vi "Clear Scan Time Out_4.vi"(6 "Channel number":i32, 7 "ESP32 ref":refnum<visa-resource-name>="COM4", 8 "error in (no error)":errorcluster, 11 "VISA Refnum in":refnum<visa-resource-name>) -> (0 "error out":errorcluster, 1 "error?":bool, 2 "Time out count":i32, 3 "VISA Refnum out":refnum<visa-resource-name>, 5 "ESP32 ref out":refnum<visa-resource-name>)   [LabVIEW 2023]
uses:
  <vilib>/Utility/error.llb/DialogType.ctl
  <instrlib>/Agilent 3446X Series/Agilent 3446X Series.lvlib
panel:
  out "error out 3":errorcluster
  out "error out 2":errorcluster
  out "s? t:f 2":bool
  out "Measurements":dbl[](array[numeric])
  out "length":i32
  out "array":dbl[](array[numeric])
  out "return count":u32
  out "Channel number 2":i32
  out "size(s)":i32
  out "x >= y?":bool
  out "s? t:f":bool
  out "Numeric":i32
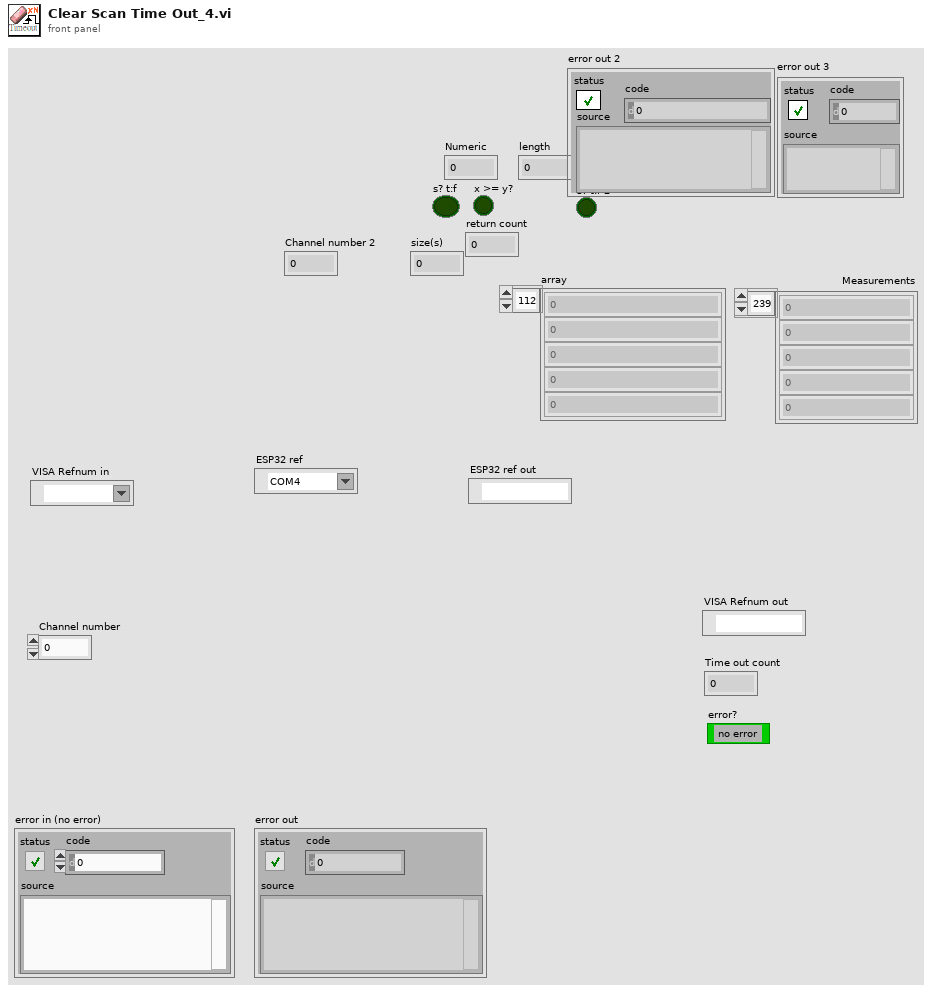
[diagram p1: front panel]
types:
  T1 = typedef "DialogType.ctl" = u16
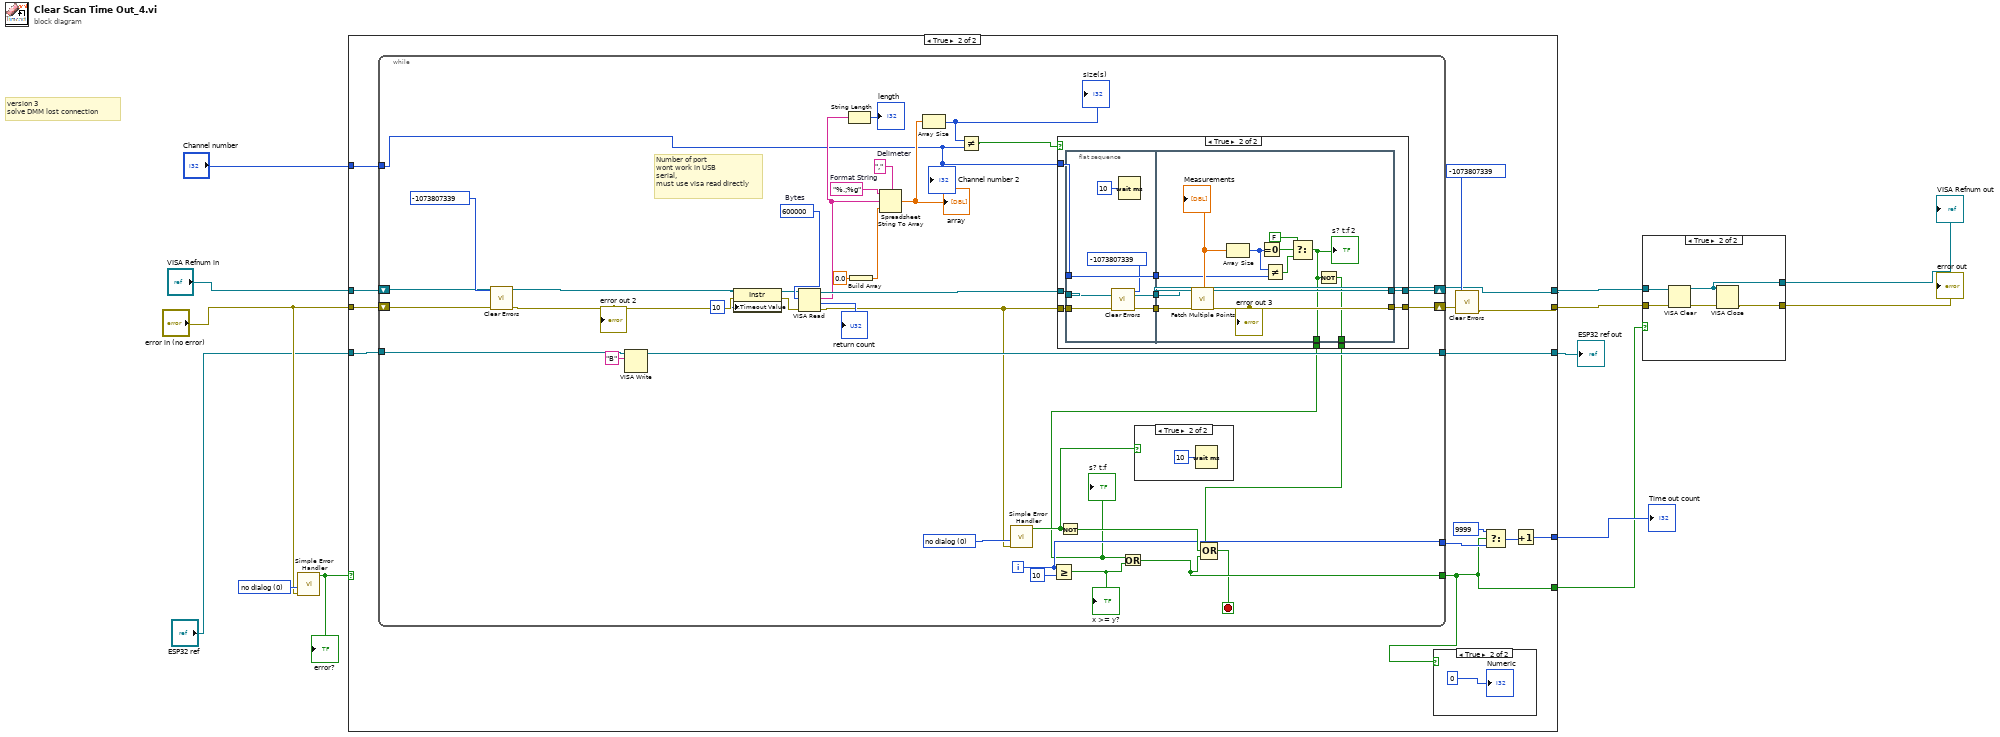
[diagram p0: block diagram]
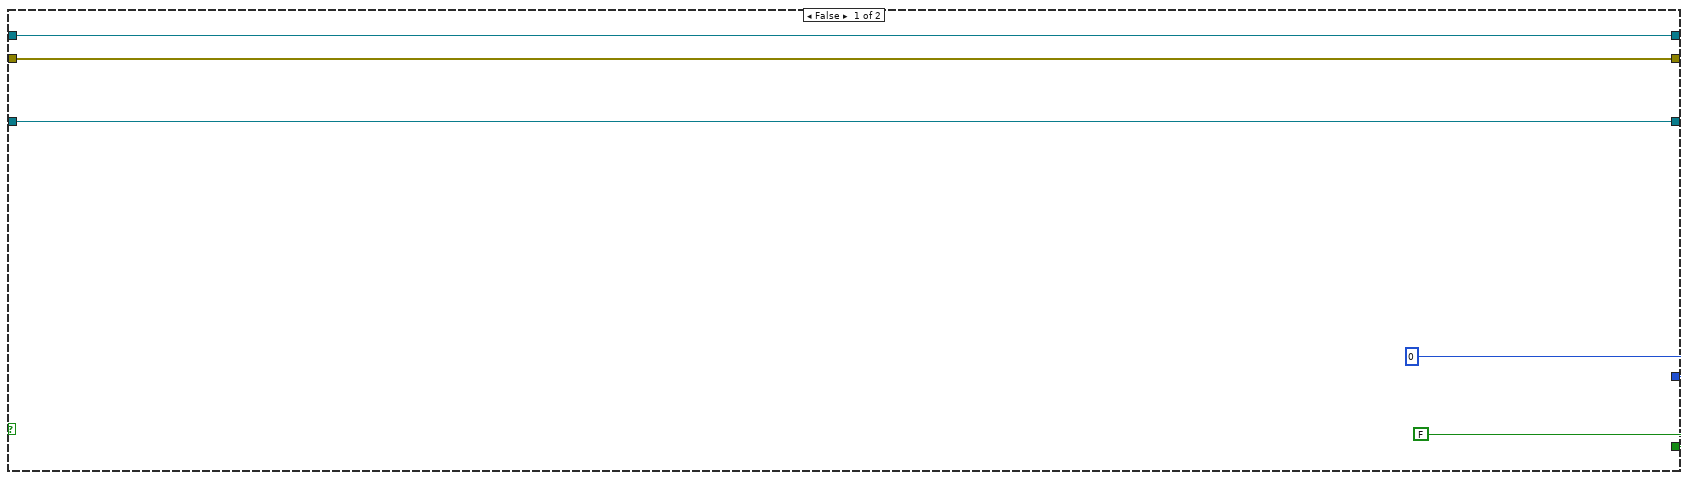
[diagram p3: hidden frame]
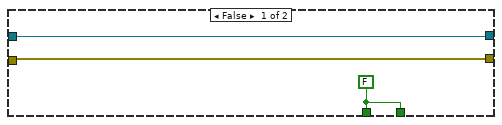
[diagram p5: hidden frame]
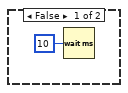
[diagram p6: hidden frame]
diagram:
  w12 = T1 0 items=["no dialog", "OK message", "continue or stop message", "OK message + warnings", "continue/stop + warnings"] ("type of dialog (OK msg:1)")
  # "version 3\nsolve DMM lost connection"
  n1 = call <vilib>:"Simple Error Handler.vi"("type of dialog (OK msg:1)"=w12, "error in (no error)"="error in (no error)") -> ("error?"=w10:bool)  [unwired: 3 in, 4 out]
  "error?" <- w10
  n2 = case shown="True" w10 {
    tunnel: [w18 w21] -> w4
    tunnel: "error in (no error)" -> [w17 w32]
    tunnel: "VISA Refnum in" -> [w18 w31]
    tunnel: [w17 w20] -> w3
    tunnel: [0 w30] -> w9
    tunnel: "ESP32 ref" -> [w16 w28]
    tunnel: [w16 w27] -> w7
    tunnel: "Channel number" -> [_ w26]
    tunnel: [FALSE w19] -> w5
    frame False {
    }
    frame True {
      n3 = while {
        shift-right: [w40] -> w25
        shift-left: w32 -> [w68]
        shift-right: [w41] -> w21
        shift-left: w31 -> [w53]
        tunnel: [w45] -> w22
        tunnel: [w49] -> w19
        tunnel: w28 -> [w52]
        tunnel: [w47] -> w27
        tunnel: w26 -> [w37]
        i -> [w45]
        stop <- w46 stop-if-true
        w60 = ","  # Delimeter
        w61 = "%.;%g"  # Format String
        w57 = u32 600000  # Bytes
        w66 = T1 0 items=["no dialog", "OK message", "continue or stop message", "OK message + warnings", "continue/stop + warnings"] ("type of dialog (OK msg:1)")
        # "Number of port\nwont work in USB \nserial,\nmust use visa read directly"
        n4 = call <vilib>:"Clear Errors.vi"("error in (no error)"=w68, "specific error code to clear (0: all)"=-1073807339 ("code out")) -> ("error out"=w67:errorcluster)  [unwired: 4 in, 1 out]
        "error out 2" <- w67
        n5 = VISA Write(VISA resource name=w52, write buffer="B") -> (VISA resource name out=w47:refnum<visa-resource-name>)  [unwired: 1 in, 2 out]
        n6 = property class="Instr"(reference=w53, error in=w67, "General Settings:Timeout Value"=u32 10) -> (reference out=w56:refnum<visa-resource-name>, error out=w55:errorcluster)
        n7 = VISA Read(VISA resource name=w56, byte count=w57, error in (no error)=w55) -> (VISA resource name out=w43:refnum<visa-resource-name>, read buffer=w39:string, return count=→"return count":u32, error out=w42:errorcluster)
        n8 = String Length(string=w39) -> (length=→"length":i32)
        n9 = Build Array(0.0) -> (w58:dbl[])
        n10 = Spreadsheet String To Array(delimiter (Tab)=w60, format string=w61, spreadsheet string=w39, array type (2D Dbl)=w58) -> (array=w51:dbl[])
        "array" <- w51
        n11 = Array Size(array=w51) -> (size(s)=w48:i32)
        "size(s)" <- w48
        n12 = Not Equal?(x=w48, y=w37) -> (x != y?=w34:bool)
        n13 = call <vilib>:"Simple Error Handler.vi"("type of dialog (OK msg:1)"=w66, "error in (no error)"=w42) -> ("error?"=w63:bool)  [unwired: 3 in, 4 out]
        n14 = Greater Or Equal?(x=w45, y=10) -> (x >= y?=w50:bool)
        "x >= y?" <- w50
        n15 = case shown="True" w34 {
          tunnel: w43 -> [w72 w79]
          tunnel: w42 -> [w71 w78]
          tunnel: [w72 w77] -> w41
          tunnel: [w71 w76] -> w40
          tunnel: w37 -> [_ w75]
          tunnel: [w70 w74] -> w36
          tunnel: [w70 w73] -> w35
          frame False {
            w70 = FALSE ("t")
          }
          frame True {
            n16 = flat-sequence {
              tunnel: w78 -> [w85]
              tunnel: w79 -> [w88]
              tunnel: [w88] -> w82
              tunnel: [w84] -> w81
              tunnel: w75 -> [w86]
              tunnel: [w86] -> w80
              tunnel: [w98] -> w77
              tunnel: [w97] -> w76
              tunnel: w82 -> [w100]
              tunnel: w81 -> [w99]
              tunnel: w80 -> [w91]
              tunnel: [w90] -> w74
              tunnel: [w89] -> w73
              frame #0 {
                n17 = call <vilib>:"Clear Errors.vi"("error in (no error)"=w85, "specific error code to clear (0: all)"=-1073807339) -> ("error out"=w84:errorcluster)  [unwired: 4 in, 1 out]
                n18 = Wait (ms)(milliseconds to wait=u32 10) -> ()  [unwired: 1 out]
              }
              frame #1 {
                n19 = call <instrlib>:"Fetch Multiple Points.vi"("error in (no error)"=w99, "VISA resource name"=w100) -> ("error out"=w97:errorcluster, "Measurements"=w92:dbl[], "VISA resource name out"=w98:refnum<visa-resource-name>)  [unwired: 7 in]
                "Measurements" <- w92
                "error out 3" <- w97
                n20 = Array Size(array=w92) -> (size(s)=w93:i32)
                n21 = Equal To 0?(x=w93) -> (x = 0?=w96:bool)
                n22 = Not Equal?(x=w93, y=w91) -> (x != y?=w95:bool)
                n23 = Select(t=FALSE, s=w96, f=w95) -> (s? t:f=w90:bool)
                "s? t:f 2" <- w90
                n24 = Not(x=w90) -> (.not. x?=w89:bool)
              }
            }
          }
        }
        "s? t:f" <- w36
        n25 = Not(x=w63) -> (.not. x?=w64:bool)
        n26 = Or(x=w36, y=w50) -> (x .or. y?=w49:bool)
        n27 = case shown="True" w63 {
          frame False {
            n28 = Wait (ms)(milliseconds to wait=u32 10) -> ()  [unwired: 1 out]
          }
          frame True {
            n29 = Wait (ms)(milliseconds to wait=u32 10) -> ()  [unwired: 1 out]
          }
        }
        n30 = Compound Arithmetic op=OR(w35, w64, w49) -> (w46:bool)
        "Channel number 2" <- w37
      }
      n31 = case shown="True" w19 {
        frame False {
        }
        frame True {
          "Numeric" <- 0
        }
      }
      n32 = call <vilib>:"Clear Errors.vi"("error in (no error)"=w25, "specific error code to clear (0: all)"=-1073807339 ("code out")) -> ("error out"=w20:errorcluster)  [unwired: 4 in, 1 out]
      n33 = Select(t=9999, s=w19, f=w22) -> (s? t:f=w29:i32)
      n34 = Increment(x=w29) -> (x+1=w30:i32)
    }
  }
  "Time out count" <- w9
  "ESP32 ref out" <- w7
  n35 = case shown="True" w5 {
    tunnel: w4 -> [w104 w108]
    tunnel: w3 -> [w103 w109]
    tunnel: [w103 w106] -> w2
    tunnel: [w104 w105] -> w1
    frame False {
    }
    frame True {
      n36 = VISA Clear(VISA resource name=w108, error in (no error)=w109) -> (VISA resource name out=w105:refnum<visa-resource-name>, error out=w107:errorcluster)
      n37 = VISA Close(VISA resource name=w105, error in (no error)=w107) -> (error out=w106:errorcluster)
    }
  }
  "error out" <- w2
  "VISA Refnum out" <- w1
